vi "PFI-28000-Chan-28144_Get Balance Mode.vi"(8 "error in (no error)":errorcluster, 11 "PFI-28000-Chan-28144 in":refnum<class "PFI-28000-Chan-28144.lvclass">) -> (0 "error out":errorcluster, 2 "Balance Mode":T1, 3 "PFI-28000-Chan-28144 out":refnum<class "PFI-28000-Chan-28144.lvclass">)   [LabVIEW 2017, in "PFI-28000-Chan-28144.lvclass"]
uses:
  PFI-28000-Chan-28144.lvclass
  C:/wc/07143 Precision Filters 28000 Support/Driver/source/Channel/PFI-28000-Channel.lvclass
  PFI-28000-Chan-28144-Balance Mode.ctl
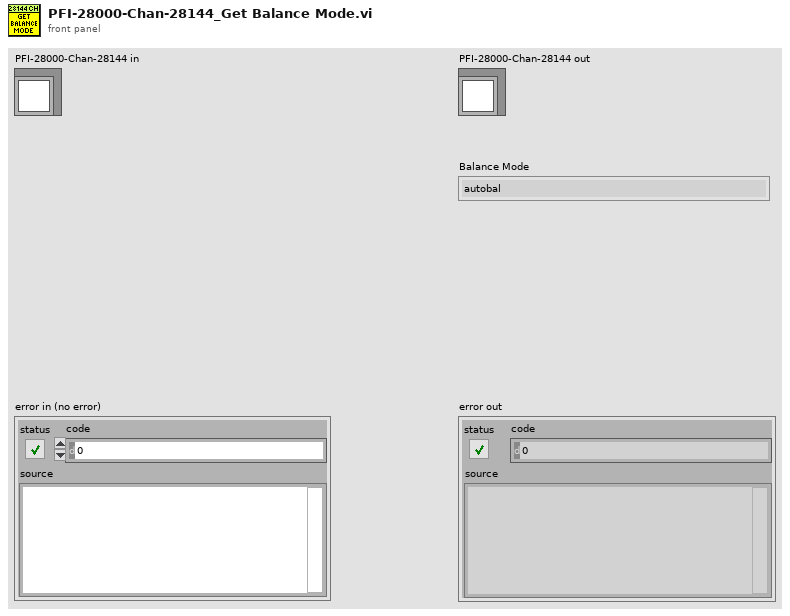
[diagram p1: front panel]
types:
  T1 = typedef "PFI-28000-Chan-28144.lvclass/PFI-28000-Chan-28144-Balance Mode.ctl" = enum8{"autobal", "zerosup"}
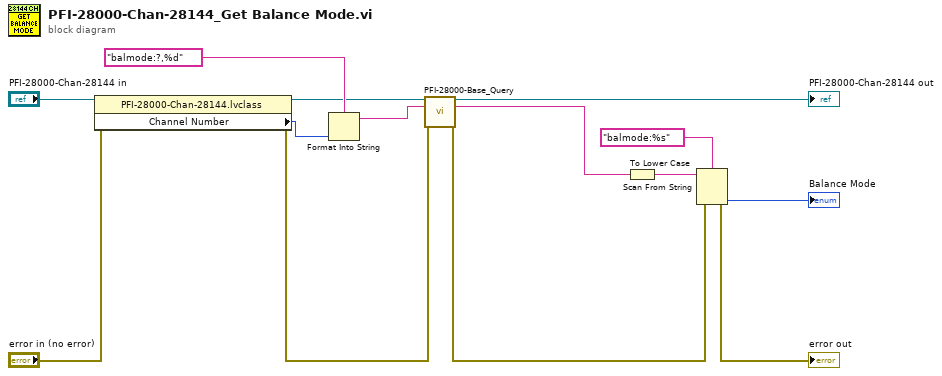
[diagram p0: block diagram]
diagram:
  n1 = property class="PFI-28000-Chan-28144.lvclass"(reference="PFI-28000-Chan-28144 in", error in="error in (no error)") -> (reference out=w6:refnum<class "PFI-28000-Chan-28144.lvclass">, error out=w2:errorcluster, "Channel Number"=w10:i32)
  n2 = Format Into String(format string="balmode:?,%d" ("empty string"), w10) -> (resulting string=w4:string)  [unwired: 2 in, 1 out]
  n3 = call-dynamic "PFI-28000-Base_Query.vi"("PFI-28000-Base in"=w6, "Command"=w4, "error in (no error)"=w2) -> ("PFI-28000-Base out"=→"PFI-28000-Chan-28144 out":refnum<class "PFI-28000-Chan-28144.lvclass">, "Response"=w3:string, "error out"=w1:errorcluster)  [unwired: 9 in, 1 out]
  n4 = To Lower Case(string=w3) -> (all lower case string=w7:string)
  n5 = Scan From String(format string="balmode:%s" ("empty string"), input string=w7, error in=w1) -> (error out=→"error out":errorcluster, output 1=→"Balance Mode":T1)  [unwired: 2 in, 2 out]
